vi "Global_CAMERA.vi"() -> ()   [LabVIEW 2015]
panel:
  out "kinetic time (s)":sgl
  out "CAMERA ready":bool
  out "Start CAMERA":bool
  out "Frames acquired":i32
  out "CAMERA done":bool
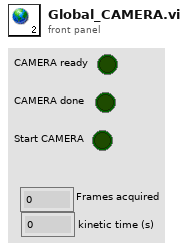
[diagram p1: front panel]
diagram:
